vi "calibrate_6dof_kinematics.vi"() -> ()   [LabVIEW 2013]
uses:
  <vilib>/Analysis/Matrix/Datatypes/RealMatrix.ctl
  <vilib>/Platform/TimedLoop/XDataNode/timing_clust.ctl
  <vilib>/Platform/TimedLoop/XDataNode/nitl_modes.ctl
  <vilib>/Platform/TimedLoop/XDataNode/wakeup.ctl
  cancellation/decoupled_gain.ctl
  testing/injection_point.ctl
  testing/probe_point.ctl
  <vilib>/Analysis/4window.llb/Hanning Window (DBL).vi
  <vilib>/Analysis/4window.llb/AllCosWindow (DBL).vi
  initialization/micron_globals.vi
  cancellation/decoupling_global.vi
  <vilib>/Analysis/baseanly.llb/Real Inverse Matrix.vi
  <vilib>/Analysis/Matrix/Numeric/Multiply/Multiply - RM,R.vi
  <vilib>/Analysis/Matrix/Numeric/Subtract/Subtract - RM,RM.vi
  <vilib>/Analysis/Matrix/Numeric/Absolute Value/Absolute Value - RM.vi
  <vilib>/Analysis/Matrix/Numeric/Conversions/Matrix To Array - RM.vi
  <vilib>/Analysis/Matrix/Numeric/Conversions/Array To Matrix - RA.vi
  <vilib>/Platform/TimedLoop/XDataNode/XDataNode.xnode
  <vilib>/Platform/TimedLoop/XDataNode/XDNodeRunTimeDep.lvlib
  <vilib>/Analysis/NI_AALBase.lvlib
  <vilib>/Analysis/NI_AALPro.lvlib
  <vilib>/Analysis/Matrix/NI_Matrix.lvlib
panel:
  in  "Use Output Enable":bool
  out "inv(Reference)":T1 format="%#.3g"
  in  "Compare ref inverse":bool
  out "Scale estimate":dbl format="%#_3p"
  in  "Scale":dbl=1.0 step=0.1 format="%#_3p"
  out "Ratio comparison":T1 format="%#.2g"
  out "RMS":dbl format="%#_3p"
  in  "Set ref":bool
  out "Reference":T1 format="%#.3g"
  out "Comparison":T1 format="%#.2g"
  in  "Bandwidth":dbl=30.0
  in  "Method":enum16{"Quasi-open", "Closed loop"}(ring)
  out "Axis permutation (row)":T1 format="%#.0f"
  out "Unpermuted":T1 format="%#.3g"
  in  "Axis permutation":i32[](array[numeric])=[0, 1, 2, 3, 4, 5]
  in  "Store":bool
  in  "Scan axes":bool[](array[boolean])=[TRUE, TRUE, TRUE, TRUE, TRUE, TRUE]
  out "Inverse":T1 format="%#.3g"
  out "From max (dB)":T1 format="%#_3g"
  out "To max (dB)":T1 format="%#_3g"
  out "Correlation results":dbl[][](graph)
  in  "Length":dbl=2.5
  out "Preprocessed signals":dbl[][](graph)
  in  "Frequency":dbl=5.0
  in  "stop":bool
  out "Coupling":T1 format="%#.3g"
  in  "Amplitude":sgl=5.0
  in  "Scanning":bool
  in  "Scan":bool
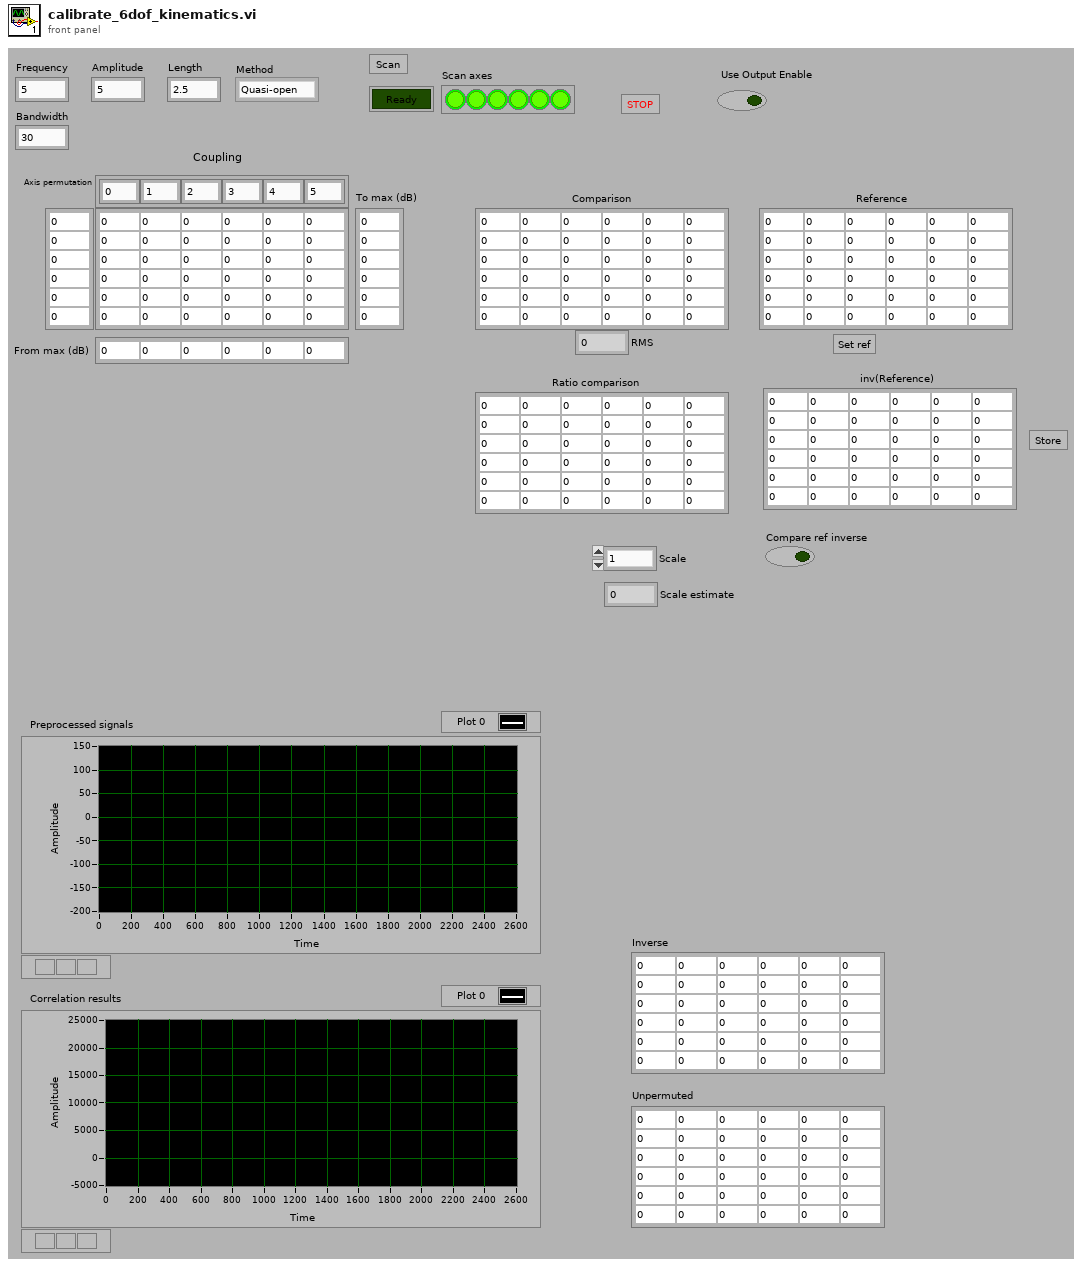
[diagram p1: front panel]
types:
  T1 = typedef "NI_Matrix.lvlib/RealMatrix.ctl" = dbl[][]
  T2 = typedef "XDNodeRunTimeDep.lvlib/timing_clust.ctl" = cluster{"Expected End [f-1]":u64, "Actual End [f-1]":u64, "Finished Late? [f-1]":bool, "Expected End [i-1]":u64, "Actual End [i-1]":u64, "Finished Late? [i-1]":bool, "Expected Start [i]":u64, "Actual Start [i]":u64, "Expected Start [f]":u64, "Actual Start [f]":u64, "Source Name":string, "Structure Name":string, "Period":i64, "Deadline":i64, "Offset":i64, "Start":i64, "Priority":i32, "Timeout":i32, "Mode":T3, "Wakeup Reason":T4, "Error":errorcluster, "Source Type":string, "Secondary Source Type":string, "Global End Time":u64, "Global Start Time":u64, "Frame Duration":u64, "Iteration Duration":u64, "Assigned CPU":i32, "I/O Scan Engine Mode":u32}
  T3 = typedef "XDNodeRunTimeDep.lvlib/nitl_modes.ctl" = enum32{"No Change", "Process missed periods, maintain original phase", "Discard missed periods, maintain original phase", "Process missed periods, ignore original phase", "Discard missed periods, ignore original phase"}
  T4 = typedef "XDNodeRunTimeDep.lvlib/wakeup.ctl" = enum32{"Normal", "Aborted", "Asynchronous wakeup", "Timing source error", "Timed loop error", "Timeout"}
  T5 = typedef "probe_point.ctl" = enum16{"Position (tip)", "Position (RCM)", "Null pos (tip)", "Null pos (RCM)", "V limiter (tip)", "V Limiter (RCM)", "Goal (tip)", "Goal (RCM)", "Link pos 0", "Link pos 1", "KF link pos 0", "KF link pos 1", "Link rate 0", "Link rate 1", "Link residue 0", "Link residue 1", "Link goal 0", "Link goal 1", "Rate limit 0", "Rate limit 1", "Link error 0", "Link error 1", "Controller 0", "Controller 1", "Output 0", "Output 1", "Drive 0", "Drive 1", "Stimulus 0", "Stimulus 1", "Trace data 0", "Trace data 1", "Analog data 0", "Analog data 1", "Status flags", "Light 0", "Light 1", "Light 2", "Light 3", "Light 4", "Light 5", "Goal origin", "Goal rotation 0", "Goal rotation 1", "Goal rotation 2", "Output origin", "Output rotation 0", "Output rotation 1", "Output rotation 2", "Handle origin", "Handle rotation 0", "Handle rotation 1", "Handle rotation 2", "Handle position", "Handle velocity", "Handle acceleration", "Handle angles", "Handle angle rates", "Handle pos residue", "Handle angle residue", "Trace length"}
  T6 = typedef "decoupled_gain.ctl" = cluster{"XY":sgl, "Rxy":sgl, "Z":sgl, "Rz":sgl}
  T7 = enum16{"Off", "Step", "Sine", "Triangle", "Arbitrary"}
  T8 = typedef "injection_point.ctl" = enum16{"Total pose", "V limiter", "Goal ", "Link position", "KF link position", "Inverse kin", "Link goal", "Link error", "Controller", "Output", "Drive", "Light"}
  T9 = typedef "Micron params.ctl" = cluster{"Stimulus":T10, "Goal Filter A":T11, "Mode controls":T12, "Manipulator type":enum16{"Current piezo", "Voltage piezo"}, "Manipulator calibration":T13, "Network":T15, "Goal Filter B":T11, "Cancellation":T16, "Transition time":sgl, "Estimation":T17}
  T10 = typedef "stimulus.ctl" = cluster{"Type":enum16{"Off", "Step", "Sine", "Triangle", "Arbitrary"}, "Phase":dbl, "Amplitude":sgl[], "Injection point":T8, "Closed loop":bool, "Offset":sgl[], "Tip -> world":bool, "Frequency":dbl, "Length":dbl}
  T11 = typedef "goal_loop_parms.ctl" = cluster{"Speedup max":sgl, "Speedup thresh":sgl, "Speedup nonlin":sgl, "Filters":cluster{"Lower Fc":sgl, "Lower Q":sgl, "Scale factor":sgl, "Upper Fc":sgl, "Upper Q":sgl, "V limit":sgl, "V limit range":sgl}[]}
  T12 = typedef "mode_conrols.ctl" = cluster{"Hold":bool, "Cancellation":bool, "Goal filter":bool, "Trigger":bool}
  T13 = typedef "manipulator_cal.ctl" = cluster{"Tool offsets":sgl[][], "Tip light calibration":T14, "Handle light calibration":T14, "Base pivots":sgl[][], "Output pivots":sgl[][], "Length center":sgl, "Workspace height":sgl[], "Workspace diameter":sgl[], "Linearization":sgl[][], "Stack travel":sgl, "Saturation pos":sgl, "Inverse filters":cluster{"filter structure":enum32{"IIR 2nd Order", "IIR 4th Order"}, "Reverse Coefficients":dbl[], "Forward Coefficients":dbl[]}[]}
  T14 = typedef "probe_calibration.ctl" = sgl[][]
  T15 = typedef "network_params.ctl" = cluster{"Remote Host":string, "Send Status":bool, "Send Port":u16, "Recv Commands":bool, "Recv Port":u16}
  T16 = typedef "sq_control_params.ctl" = cluster{"KP":T6, "KI":sgl, "KD":T6, "Max vel":sgl, "Max acc":sgl, "Int error limit":sgl, "RCM gain":sgl, "Bypass":bool, "Degraded gain":sgl}
  T17 = typedef "estimation_controls.ctl" = cluster{"Link":cluster{"Measure noise":dbl[], "Process noise":dbl[], "Alt process noise":dbl[], "Alt turnoff cycles":i32, "Innovation limit":dbl[], "Residue threshold":dbl, "Enable":bool}, "Handle":cluster{"Measure noise":dbl[], "Process noise":dbl[], "State limits":dbl[], "Innovation limit":dbl[], "Prediction Lookahead":sgl, "Enable":bool}}
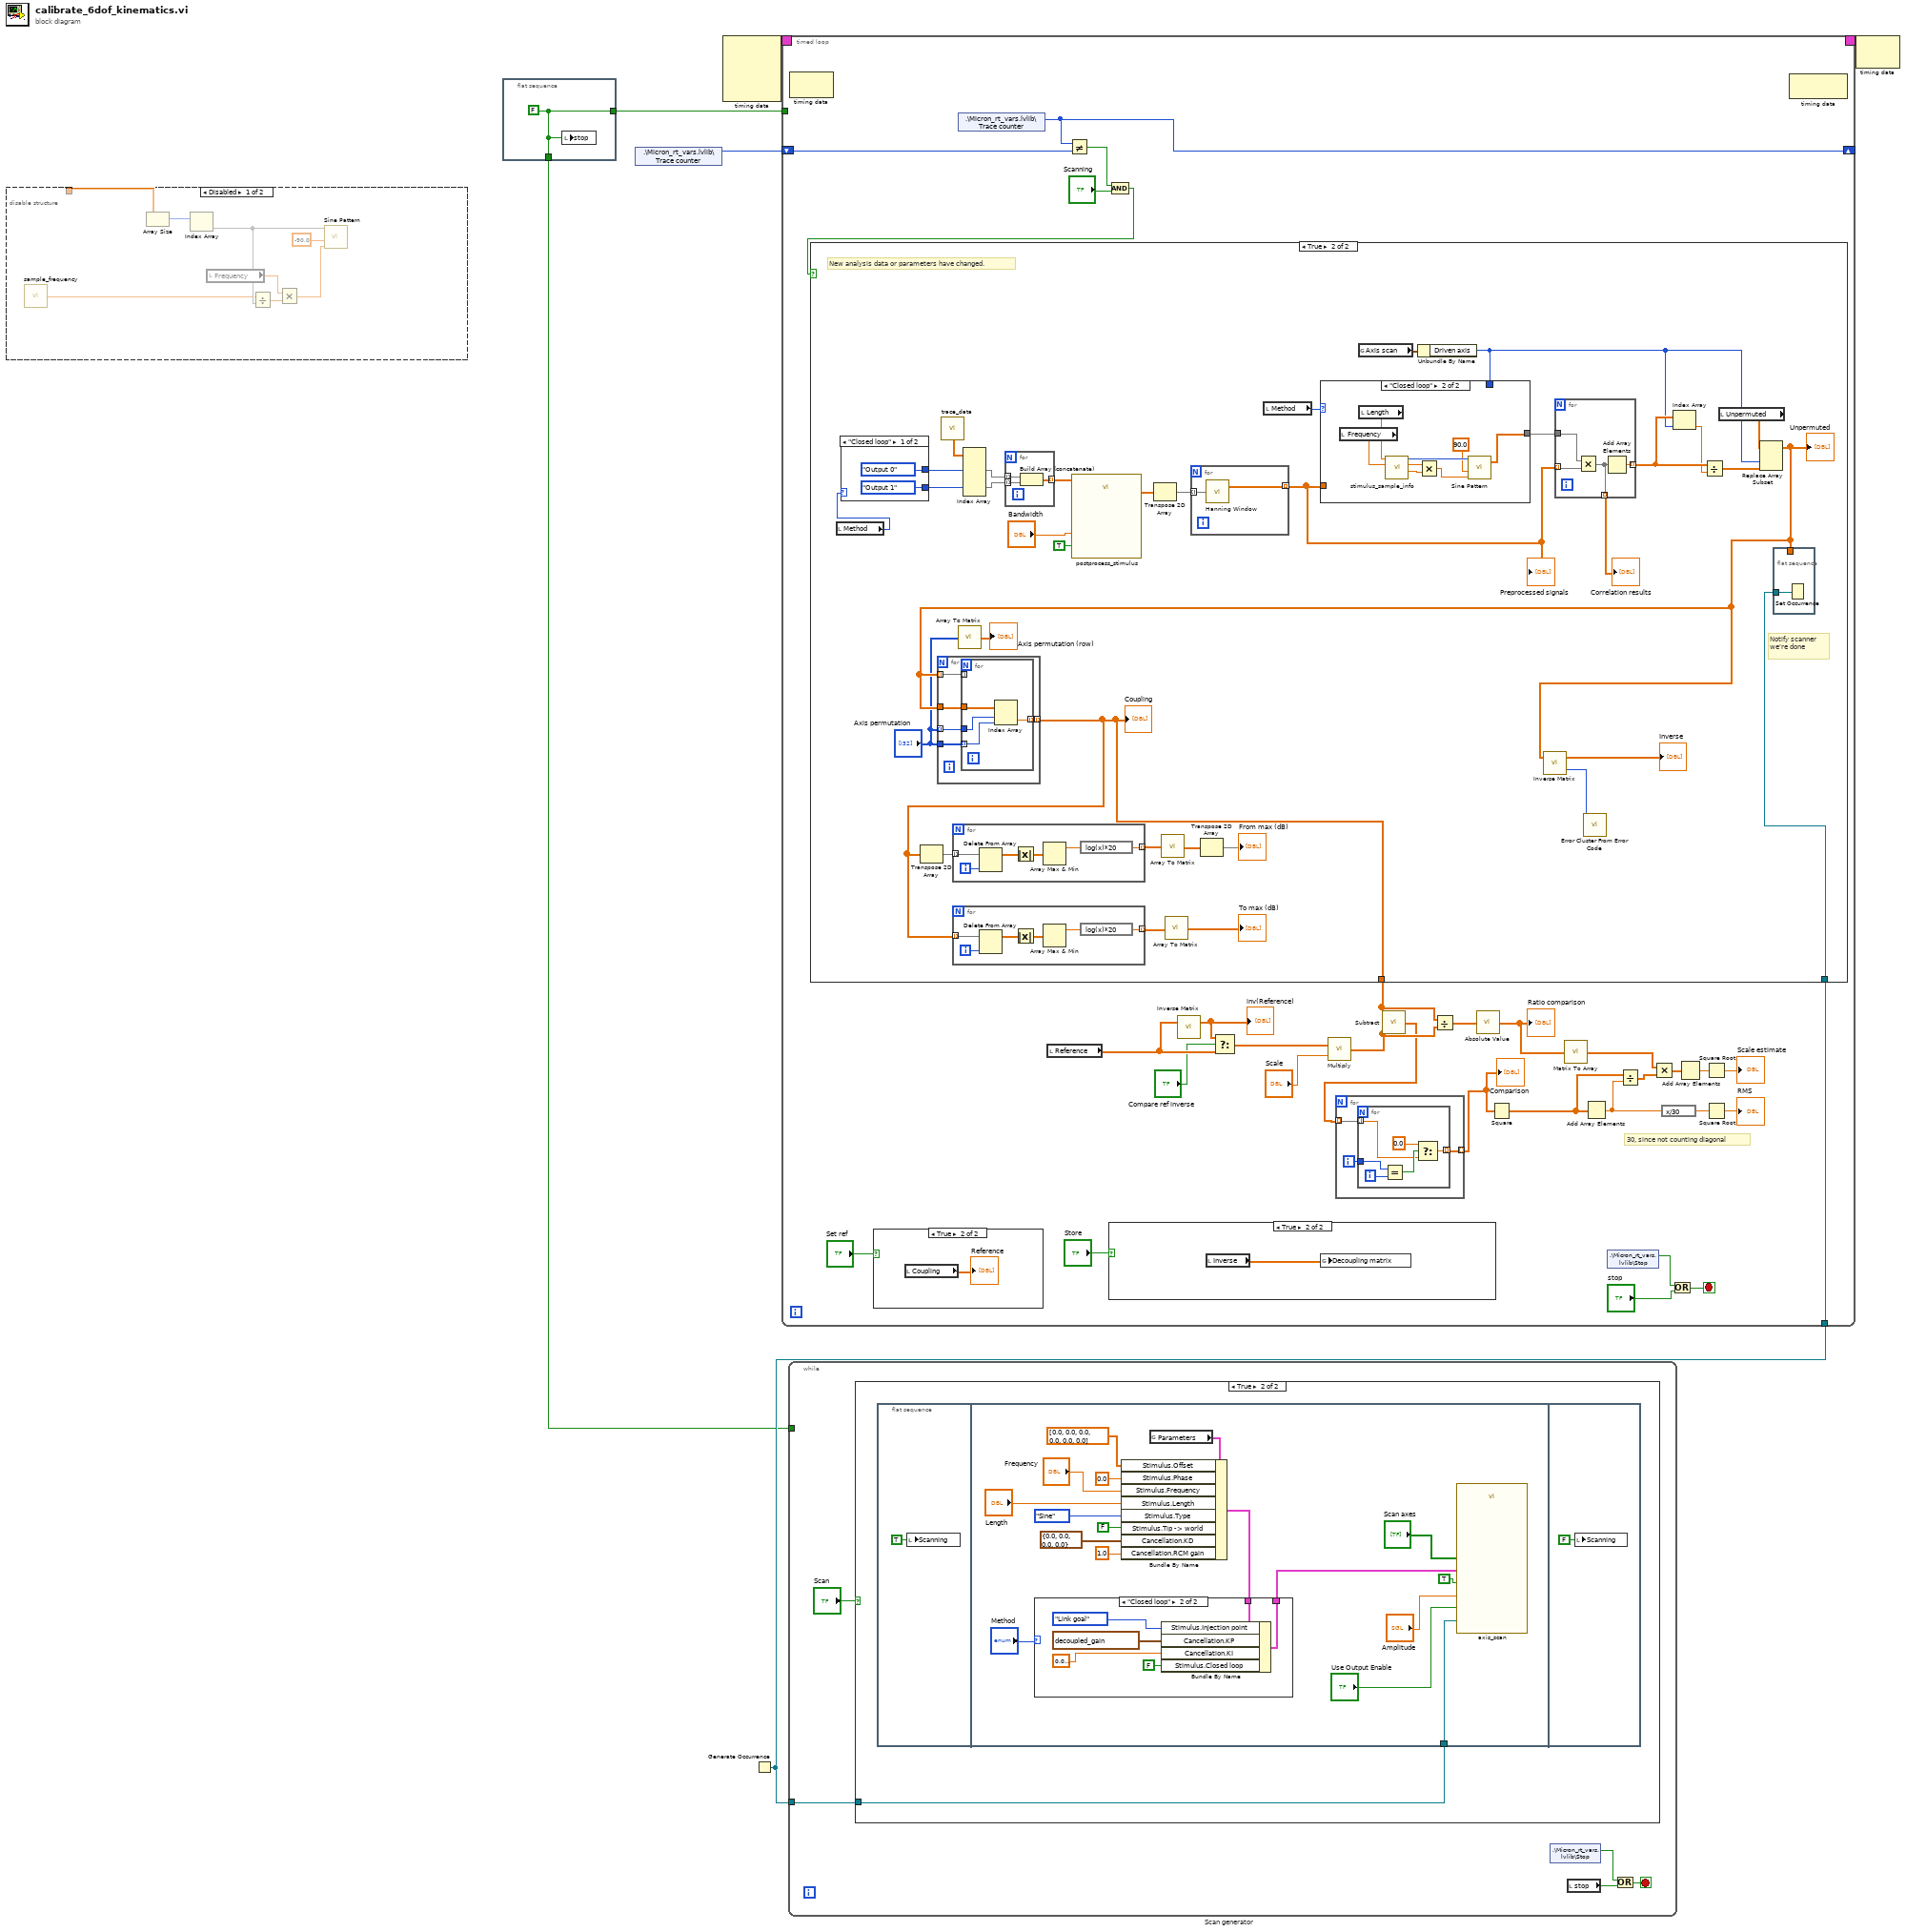
[diagram p0: block diagram]
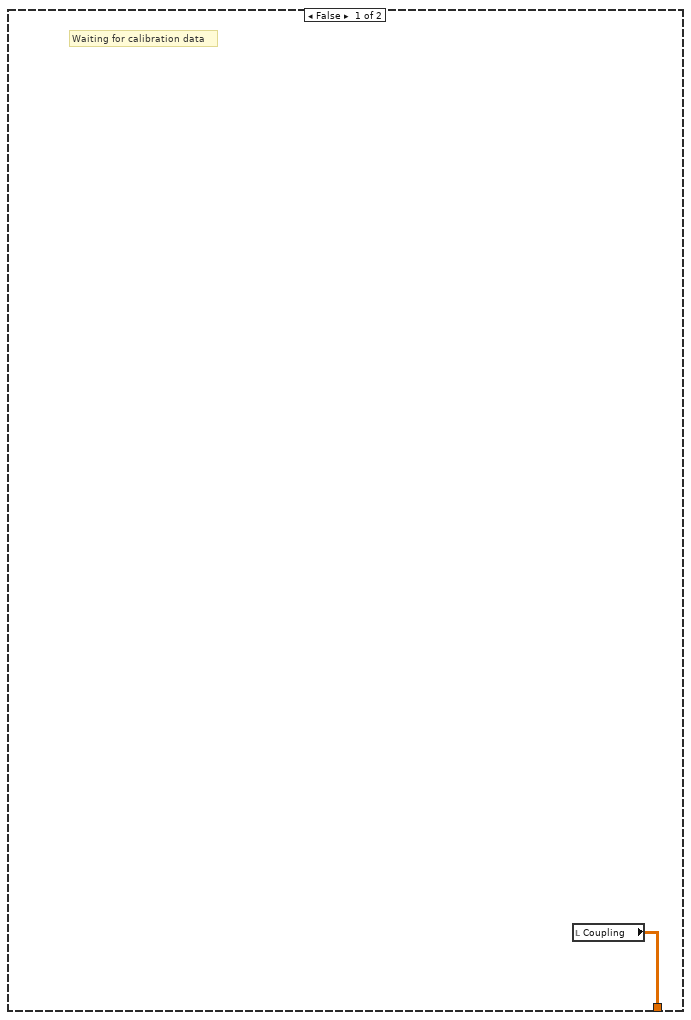
[diagram p5: hidden frame]
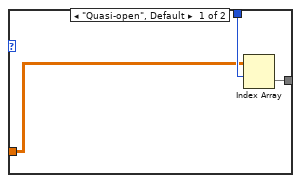
[diagram p6: hidden frame]
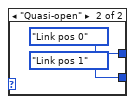
[diagram p7: hidden frame]
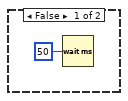
[diagram p8: hidden frame]
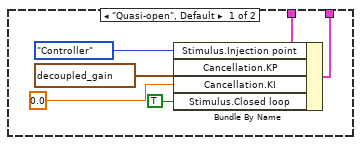
[diagram p9: hidden frame]
diagram:
  n1 = disable-structure shown="Disabled" {
    disable-tunnel: _ -> [w14 _]
    frame Disabled {
      n2 = call "sample_frequency.vi"() -> ("Sample frequency"=w10:dbl)
      n3 = Array Size(array=w14) -> (size(s)=w13:i32)
      n4 = Index Array(array=w13) -> (element=w11)  [unwired: 1 in]
      n5 = local read "Frequency"() -> (w8:dbl)
      n6 = Divide(x=w10, y=w11) -> (x/y=w9:dbl)
      n7 = Multiply(x=w8, y=w9) -> (x*y=w7:dbl)
      n8 = call <vilib>:"Sine Pattern.vi"("cycles"=w7, "phase(degrees)"=-90.0, "samples"=w11) -> ()  [unwired: 1 in, 2 out]
    }
    frame Enabled {
    }
  }
  n9 = flat-sequence {
    tunnel: [w15] -> w2
    tunnel: [w15] -> w1
    frame #0 {
      w15 = FALSE ("stop")
      n10 = local write "stop"(w15) -> ()
    }
  }
  n11 = shared-variable ".\\Micron_rt_vars.lvlib\\Trace counter"() -> (w4:u32)  [unwired: 2 out]
  n12 = node-c288() -> (w6:T2)  [unwired: 4 out]
  n13 = Generate Occurrence() -> (w3:refnum<k4>)
  n14 = timed-loop {
    timing: w6 -> [_]
    timing-out: [_] -> w5
    shift-right: [w45] -> _
    shift-left: w4 -> [w46]
    tunnel: w3 -> [w41]
    tunnel: w2 -> [_]
    stop <- w42 stop-if-true
    # "30, since not counting diagonal"
    n15 = node-c288() -> ()  [unwired: 2 out]
    n16 = case shown="True" "Set ref" {
      frame False {
      }
      frame True {
        n17 = local read "Coupling"() -> (→"Reference":T1)
      }
    }
    n18 = shared-variable ".\\Micron_rt_vars.lvlib\\Trace counter"() -> (w45:u32)  [unwired: 2 out]
    n19 = local read "Reference"() -> (w21:T1)
    n20 = Not Equal?(x=w45, y=w46) -> (x != y?=w39:bool)
    n21 = And(x=w39, y="Scanning") -> (x .and. y?=w38:bool)
    n22 = case shown="True" w38 {
      tunnel: w41 -> [_ w88]
      tunnel: [w58 w59] -> w35
      frame False {
        # "Waiting for calibration data"
        n23 = local read "Coupling"() -> (w58:T1)
      }
      frame True {
        # "Notify scanner we're done"
        # "New analysis data or parameters have changed."
        n24 = local read "Method"() -> (w65:enum16{"Quasi-open", "Closed loop"})
        n25 = case shown="\"Closed loop\"" w65 {
          tunnel: [probe_point."Output 0" ("Probe point") probe_point."Link pos 0" ("Probe point")] -> w92
          tunnel: [probe_point."Output 1" ("Probe point") probe_point."Link pos 1" ("Probe point")] -> w91
          frame "Closed loop" {
          }
          frame "Quasi-open" {
          }
        }
        n26 = call "trace_data.vi"() -> ("Decimated trace"=w87:sgl[][][])  [unwired: 9 in, 2 out]
        n27 = call-poly <vilib>:"Array To Matrix.vi"("Real 1D Array"="Axis permutation") -> ("Real Matrix (Column Vector)"=→"Axis permutation (row)":T1)
        n28 = Index Array(array=w87, index (dim 1) #1=w92, index (dim 1) #2=w91) -> (element #1=w90:sgl[][], element #2=w89:sgl[][])  [unwired: 4 in]
        n29 = for {
          tunnel: w90 -> [w139] mode=indexing
          tunnel: w89 -> [w138] mode=indexing
          tunnel: [w137] -> w79 mode=indexing
          n30 = Build Array (concatenate)(w139, w138) -> (w137:sgl[])
        }
        n31 = call "postprocess_stimulus.vi"("Bandwidth"="Bandwidth", "Detrend"=TRUE, "Input"=w79) -> ("Output"=w80:sgl[][])  [unwired: 8 in]
        n32 = Transpose 2D Array(2D array=w80) -> (transposed array=w61:sgl[][])
        n33 = for {
          tunnel: w61 -> [w94] mode=indexing
          tunnel: [w93] -> w60 mode=indexing
          n34 = call-poly <vilib>:"Hanning Window.vi"("X"=w94) -> ("Windowed X"=w93:dbl[])  [unwired: 1 out]
        }
        "Preprocessed signals" <- w60
        n35 = local read "Method"() -> (w64:enum16{"Quasi-open", "Closed loop"})
        n36 = global read "micron_globals.vi" "Axis scan"() -> (w86:cluster{"Driven axis":i32, "Scan index":i32})
        n37 = Unbundle By Name(w86) -> ("Driven axis"=w63:i32)
        n38 = case shown="\"Closed loop\"" w64 {
          tunnel: w60 -> [w95 _]
          tunnel: w63 -> [w97 _]
          tunnel: [w96 w98] -> w62
          frame "Quasi-open", Default {
            n39 = Index Array(array=w95, index (row)=w97) -> (element=w96:dbl[])  [unwired: 1 in]
          }
          frame "Closed loop" {
            n40 = local read "Frequency"() -> (w105:dbl)
            n41 = local read "Length"() -> (w104:dbl)
            n42 = call "stimulus_sample_info.vi"("Frequency"=w105, "Length"=w104) -> ("Actual frequency"=w101:dbl, "Actual length"=w102:dbl, "Num samples"=w103:i32)  [unwired: 6 in, 1 out]
            n43 = Multiply(x=w102, y=w101) -> (x*y=w100:dbl)
            n44 = call <vilib>:"Sine Pattern.vi"("cycles"=w100, "phase(degrees)"=90.0, "samples"=w103) -> ("Sinusoidal Pattern"=w98:dbl[])  [unwired: 1 in, 1 out]
          }
        }
        n45 = for {
          tunnel: w60 -> [w135] mode=indexing
          tunnel: [w134] -> w84 mode=indexing
          tunnel: [w133] -> w77 mode=indexing
          tunnel: w62 -> [w132]
          n46 = Multiply(x=w132, y=w135) -> (x*y=w133:dbl[])
          n47 = Add Array Elements(numeric array=w133) -> (sum=w134:dbl)
        }
        "Correlation results" <- w77
        n48 = Index Array(array=w84, index=w63) -> (element=w83:dbl)
        n49 = Divide(x=w84, y=w83) -> (x/y=w78:dbl[])
        n50 = local read "Unpermuted"() -> (w85:T1)
        n51 = Replace Array Subset(array=w85, new element=w78, index (col)=w63) -> (w68:T1)  [unwired: 1 in]
        "Unpermuted" <- w68
        n52 = for {
          tunnel: w68 -> [w114] mode=indexing
          tunnel: w68 -> [w113]
          tunnel: "Axis permutation" -> [w112]
          tunnel: "Axis permutation" -> [w111] mode=indexing
          tunnel: [w110] -> w59 mode=indexing
          n53 = for {
            tunnel: [w119] -> _ mode=indexing
            tunnel: w114 -> [w119] mode=indexing
            tunnel: w113 -> [w118]
            tunnel: w112 -> [w116] mode=indexing
            tunnel: w111 -> [w117]
            tunnel: [w115] -> w110 mode=indexing
            n54 = Index Array(array=w118, index (row)=w117, index (col)=w116) -> (element=w115:dbl)
          }
        }
        "Coupling" <- w59
        n55 = Transpose 2D Array(2D array=w59) -> (transposed array=w72:dbl[][])
        n56 = for {
          tunnel: w72 -> [w129] mode=indexing
          tunnel: [w130] -> w76 mode=indexing
          i -> [w128]
          n57 = Delete From Array(array=w129, index=w128) -> (array with subset deleted=w127:dbl[])  [unwired: 1 in, 1 out]
          n58 = Absolute Value(x=w127) -> (abs(x)=w131:dbl[])
          n59 = Array Max & Min(array=w131) -> (max value=w126:dbl)  [unwired: 3 out]
          n60 = expression code="log(x)*20"(w126) -> (w130:dbl)
        }
        n61 = for {
          tunnel: w59 -> [w122] mode=indexing
          tunnel: [w123] -> w75 mode=indexing
          i -> [w121]
          n62 = Delete From Array(array=w122, index=w121) -> (array with subset deleted=w120:dbl[])  [unwired: 1 in, 1 out]
          n63 = Absolute Value(x=w120) -> (abs(x)=w125:dbl[])
          n64 = Array Max & Min(array=w125) -> (max value=w124:dbl)  [unwired: 3 out]
          n65 = expression code="log(x)*20"(w124) -> (w123:dbl)
        }
        n66 = call-poly <vilib>:"Array To Matrix.vi"("Real 1D Array"=w76) -> ("Real Matrix (Column Vector)"=w71:T1)
        n67 = call-poly <vilib>:"Array To Matrix.vi"("Real 1D Array"=w75) -> ("Real Matrix (Column Vector)"=→"To max (dB)":T1)
        n68 = Transpose 2D Array(2D array=w71) -> (transposed array=→"From max (dB)":T1)
        n69 = call-poly <vilib>:"Inverse Matrix.vi"("Input Matrix"=w68) -> ("error"=w74:i32, "Inverse Matrix"=→"Inverse":T1)  [unwired: 1 in]
        n70 = call <vilib>:"Error Cluster From Error Code.vi"("error code (0)"=w74) -> ()  [unwired: 8 in, 1 out]
        n71 = flat-sequence {
          tunnel: w88 -> [w136]
          tunnel: w68 -> [_]
          frame #0 {
            n72 = Set Occurrence(w136) -> ()
          }
        }
      }
    }
    n73 = case shown="True" "Store" {
      frame False {
      }
      frame True {
        n74 = local read "Inverse"() -> (w57:T1)
        n75 = global write "decoupling_global.vi" "Decoupling matrix"(w57) -> ()
      }
    }
    n76 = call-poly <vilib>:"Inverse Matrix.vi"("Input Matrix"=w21) -> ("Inverse Matrix"=w16:T1)  [unwired: 1 in, 1 out]
    "inv(Reference)" <- w16
    n77 = Select(t=w16, s="Compare ref inverse", f=w21) -> (s? t:f=w19:T1)
    n78 = call-poly <vilib>:"Multiply.vi"("Real Scalar c"="Scale", "Real Matrix A"=w19) -> ("A * c"=w34:T1)
    n79 = call-poly <vilib>:"Subtract.vi"("Real Matrix B"=w34, "Real Matrix A"=w35) -> ("A - B"=w32:T1)
    n80 = for {
      tunnel: w32 -> [w49] mode=indexing
      tunnel: [w47] -> w31 mode=indexing
      i -> [w48]
      n81 = for {
        tunnel: w49 -> [w52] mode=indexing
        tunnel: w48 -> [w54]
        tunnel: [w50] -> w47 mode=indexing
        i -> [w55]
        n82 = Equal?(x=w54, y=w55) -> (x = y?=w53:bool)
        n83 = Select(t=0.0, s=w53, f=w52) -> (s? t:f=w50:dbl)
      }
    }
    "Comparison" <- w31
    n84 = Divide(x=w35, y=w34) -> (x/y=w18:T1)
    n85 = call-poly <vilib>:"Absolute Value.vi"("Real Matrix A"=w18) -> ("|A|"=w17:T1)
    "Ratio comparison" <- w17
    n86 = Square(x=w31) -> (x^2=w26:dbl[][])
    n87 = call-poly <vilib>:"Matrix To Array.vi"("Real Matrix"=w17) -> ("Real 2D Array"=w28:dbl[][])
    n88 = Add Array Elements(numeric array=w26) -> (sum=w27:dbl)
    n89 = shared-variable ".\\Micron_rt_vars.lvlib\\Stop"() -> (w44:bool)  [unwired: 2 out]
    n90 = Divide(x=w26, y=w27) -> (x/y=w25:dbl[][])
    n91 = Multiply ("Multiply.vi")(x=w28, y=w25) -> (x*y=w24:dbl[][])
    n92 = expression code="x/30"(w27) -> (w30:dbl)
    n93 = Or(x=w44, y="stop") -> (x .or. y?=w42:bool)
    n94 = Add Array Elements(numeric array=w24) -> (sum=w23:dbl)
    n95 = Square Root(x=w23) -> (sqrt(x)=→"Scale estimate":dbl)
    n96 = Square Root(x=w30) -> (sqrt(x)=→"RMS":dbl)
    n97 = node-c288() -> ()  [unwired: 2 out]
  }
  n98 = while "Scan generator" {
    tunnel: w3 -> [w145]
    tunnel: w1 -> [_]
    stop <- w143 stop-if-true
    n99 = case shown="True" "Scan" {
      tunnel: w145 -> [_ w148]
      frame False {
        n100 = Wait (ms)(milliseconds to wait=u32 50) -> ()  [unwired: 1 out]
      }
      frame True {
        n101 = flat-sequence {
          tunnel: w148 -> [w160]
          frame #0 {
            n102 = local write "Scanning"(TRUE ("Scanning")) -> ()
          }
          frame #1 {
            n103 = global read "micron_globals.vi" "Parameters"() -> (w163:T9)
            n104 = Bundle By Name(cluster=w163, "Stimulus.Offset"=sgl[] [0.0, 0.0, 0.0, 0.0, 0.0, 0.0], "Stimulus.Phase"=0.0, "Stimulus.Frequency"="Frequency", "Stimulus.Length"="Length", "Stimulus.Type"=T7."Sine" ("Type"), "Stimulus.Tip -> world"=FALSE, "Cancellation.KD"=T6 {"XY"=0.0, "Rxy"=0.0, "Z"=0.0, "Rz"=0.0}, "Cancellation.RCM gain"=sgl 1.0) -> (w153:T9)
            n105 = case shown="\"Closed loop\"" "Method" {
              tunnel: w153 -> [w170 w177]
              tunnel: [w169 w175] -> w152
              frame "Quasi-open", Default {
                n106 = Bundle By Name(cluster=w170, "Stimulus.Injection point"=injection_point."Controller", "Cancellation.KP"=T6 {"XY"=0.005, "Rxy"=0.005, "Z"=0.005, "Rz"=0.005}, "Cancellation.KI"=sgl 0.0, "Stimulus.Closed loop"=TRUE) -> (w169:T9)
              }
              frame "Closed loop" {
                n107 = Bundle By Name(cluster=w177, "Stimulus.Injection point"=injection_point."Link goal", "Cancellation.KP"=T6 {"XY"=0.15, "Rxy"=0.15, "Z"=0.07, "Rz"=0.02}, "Cancellation.KI"=sgl 0.005 ("Cancellation.KP"), "Stimulus.Closed loop"=FALSE) -> (w175:T9)
              }
            }
            n108 = call "axis_scan.vi"("Parameters"=TRUE, "Parameters in"=w152, "Next scan occurrence"=w160, "Use Output Enable"="Use Output Enable", "Amplitude"="Amplitude", "Scan axes"="Scan axes") -> ()  [unwired: 5 in, 1 out]
          }
          frame #2 {
            n109 = local write "Scanning"(FALSE ("Scanning")) -> ()
          }
        }
      }
    }
    n110 = shared-variable ".\\Micron_rt_vars.lvlib\\Stop"() -> (w142:bool)  [unwired: 2 out]
    n111 = local read "stop"() -> (w144:bool)
    n112 = Or(x=w142, y=w144) -> (x .or. y?=w143:bool)
  }
  n113 = node-c288(w5) -> ()  [unwired: 1 out]
